vi "send_AMKSetpoint.vi"(6 "Active":bool, 7 "ID":u32=389 format="%x", 8 "Error in":errorcluster, 10 "Message":T4 {"AMK_Targetvelocity" scale=0.0..21500.0; "AMK_TorqueLimitPositive" scale=0.0..2140.0; "AMK_TorqueLimitNegative" scale=0.0..-2140.0}, 11 "ObjHandle in":T3) -> (0 "Error out":errorcluster, 3 "ObjHandle out":T3)   [LabVIEW 2017]
uses:
  <vilib>/nican/nican.llb/xobjhandle.ctl
  <vilib>/nican/nican.llb/CanFrameTimed.ctl
panel:
  in  "200/freq":i32=4
  in  "Counter":i32
  in  "CAN ID":u32=560 format="%x"
  in  "CAN frame":T1[](array[typedef]) {"Data" format="%.0x"; "ArbitrationId" format="%.0x"; "Timestamp" format="%<%I:%M:%S%3u %p\n%m/%d/%Y>T"}
  out "CAN frame out":T1[](array[typedef]) {"Data" format="%.0x"; "ArbitrationId" format="%.0x"; "Timestamp" format="%<%I:%M:%S%3u %p\n%m/%d/%Y>T"}
  in  "Message 2":T2 {"APPS2" scale=0.0..100.0; "APPS1" scale=0.0..100.0; "Steering Angle 2" scale=90.0..-90.0; "Steering Angle 1" scale=90.0..-90.0}
  in  "Active 2":bool
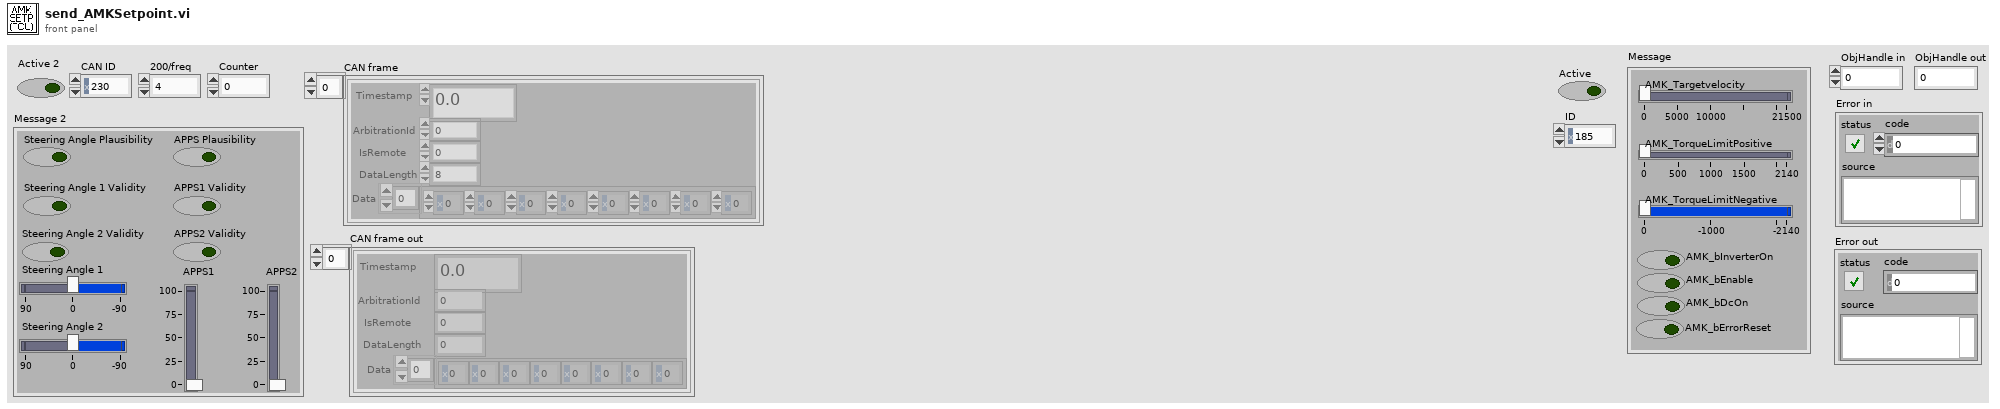
[diagram p1: front panel]
types:
  T1 = typedef "CanFrameTimed.ctl" = cluster{"Timestamp":dbl, "ArbitrationId":u32, "IsRemote":u8, "DataLength":u8, "Data":u8[]}
  T2 = cluster{"APPS Plausibility":bool, "Steering Angle 1":dbl, "Steering Angle 2":dbl, "APPS1":dbl, "APPS2":dbl, "APPS1 Validity":bool, "APPS2 Validity":bool, "Steering Angle Plausibility":bool, "Steering Angle 1 Validity":bool, "Steering Angle 2 Validity":bool}
  T3 = typedef "xobjhandle.ctl" = u32
  T4 = cluster{"AMK_bErrorReset":bool, "AMK_bDcOn":bool, "AMK_bEnable ":bool, "AMK_bInverterOn":bool, "AMK_TorqueLimitNegative":dbl, "AMK_TorqueLimitPositive":dbl, "AMK_Targetvelocity":dbl}
  T5 = cluster{"Byte 0":u8, "Byte 1":u8, "Byte 2":u8, "Byte 3":u8, "Byte 4":u8, "Byte 5":u8, "Byte 6":u8, "Byte 7":u8}
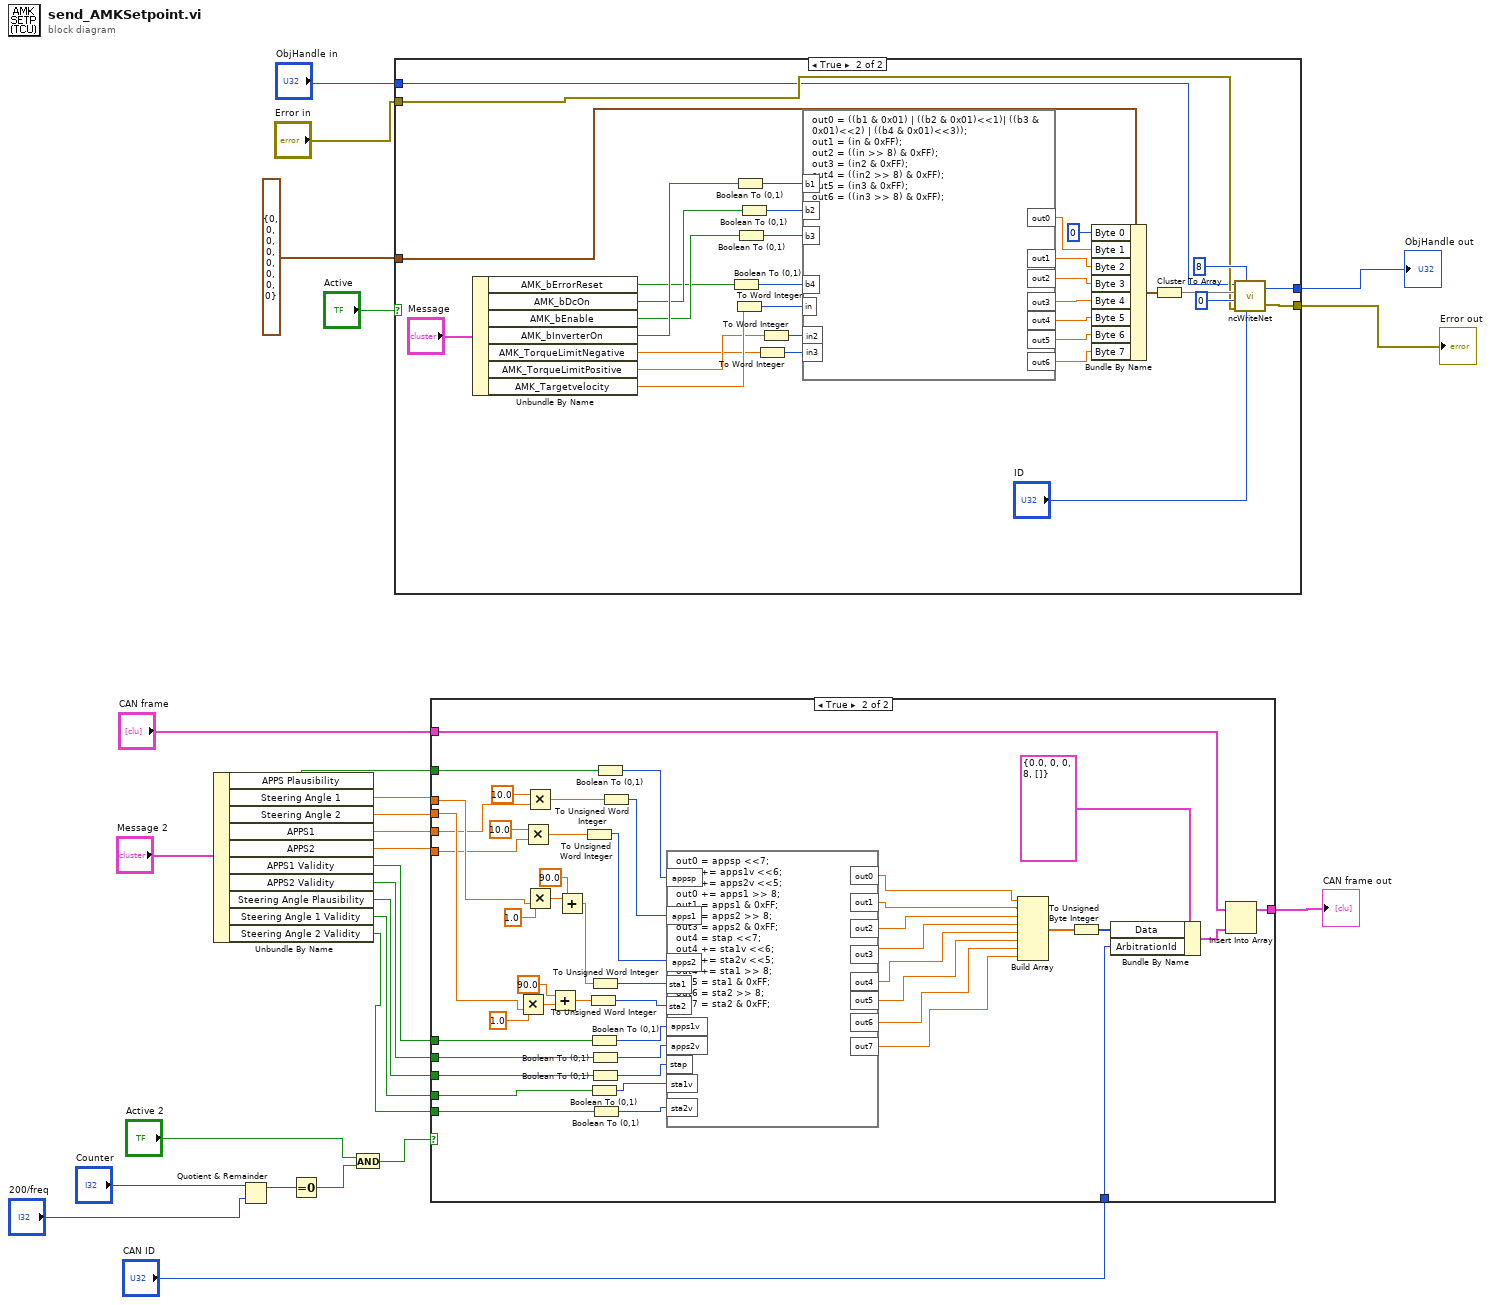
[diagram p0: block diagram]
diagram:
  n1 = Unbundle By Name("Message 2") -> ("APPS Plausibility"=w15:bool, "Steering Angle 1"=w18:dbl, "Steering Angle 2"=w19:dbl, "APPS1"=w17:dbl, "APPS2"=w16:dbl, "APPS1 Validity"=w14:bool, "APPS2 Validity"=w12:bool, "Steering Angle Plausibility"=w13:bool, "Steering Angle 1 Validity"=w11:bool, "Steering Angle 2 Validity"=w10:bool)
  n2 = Quotient & Remainder(x="Counter", y="200/freq") -> (x-y*floor(x/y)=w5:i32)  [unwired: 1 out]
  n3 = Equal To 0?(x=w5) -> (x = 0?=w3:bool)
  n4 = And(x="Active 2", y=w3) -> (x .and. y?=w2:bool)
  n5 = case shown="True" "Active" {
    tunnel: [w28 w41] -> w22
    tunnel: [w27 w40] -> w23
    tunnel: "Error in" -> [w28 w39]
    tunnel: T5 {"Byte 0"=0, "Byte 1"=0, "Byte 2"=0, "Byte 3"=0, "Byte 4"=0, "Byte 5"=0, "Byte 6"=0, "Byte 7"=0} ("CAN message") -> [_ w38]
    tunnel: "ObjHandle in" -> [w27 w37]
    frame False {
    }
    frame True {
      n6 = Unbundle By Name("Message") -> ("AMK_bErrorReset"=w32:bool, "AMK_bDcOn"=w34:bool, "AMK_bEnable"=w33:bool, "AMK_bInverterOn"=w35:bool, "AMK_TorqueLimitNegative"=w29:dbl, "AMK_TorqueLimitPositive"=w30:dbl, "AMK_Targetvelocity"=w31:dbl)
      n7 = Boolean To (0,1)(Boolean=w32) -> (0, 1=w50:i16)
      n8 = To Word Integer(number=w31) -> (16bit integer=w51:i16)
      n9 = Boolean To (0,1)(Boolean=w35) -> (0, 1=w47:i16)
      n10 = Boolean To (0,1)(Boolean=w33) -> (0, 1=w49:i16)
      n11 = Boolean To (0,1)(Boolean=w34) -> (0, 1=w48:i16)
      n12 = To Word Integer(number=w29) -> (16bit integer=w53:i16)
      n13 = To Word Integer(number=w30) -> (16bit integer=w52:i16)
      n14 = formula code="out0 = ((b1 & 0x01) | ((b2 & 0x01)<<1)| ((b3 & 0x01)<<2) | ((b4 & 0x01)<<3)); \nout1 = (in & 0xFF);\nout2 = ((in >> 8) & 0xFF);\nout3 = (in2 & 0xFF);\nout4 = ((in2 >> 8) & 0xFF);\nout5 = (in3 & 0xFF);\nout6 = ((in3 >> 8) & 0xFF);"("in"=w51, "in2"=w52, "in3"=w53, "b1"=w47, "b2"=w48, "b3"=w49, "b4"=w50) -> ("out1"=w54:dbl, "out2"=w55:dbl, "out3"=w56:dbl, "out4"=w57:dbl, "out5"=w58:dbl, "out6"=w59:dbl, "out0"=w60:dbl)
      n15 = Bundle By Name(cluster=w38, "Byte 0"=u8 0, "Byte 1"=w60, "Byte 2"=w54, "Byte 3"=w55, "Byte 4"=w56, "Byte 5"=w57, "Byte 6"=w58, "Byte 7"=w59) -> (w45:T5)
      n16 = Cluster To Array(cluster=w45) -> (array=w46:u8[])
      n17 = call <vilib>:"ncWriteNet.vi"("ArbitrationId"="ID", "DataLength"=u32 8, "Error in"=w39, "IsRemote"=u8 0, "Data"=w46, "ObjHandle in"=w37) -> ("Error out"=w41:errorcluster, "ObjHandle out"=w40:T3)
    }
  }
  "ObjHandle out" <- w23
  "Error out" <- w22
  n18 = case shown="True" w2 {
    tunnel: w19 -> [_ w93]
    tunnel: w18 -> [_ w92]
    tunnel: w17 -> [_ w91]
    tunnel: w16 -> [_ w90]
    tunnel: w15 -> [_ w89]
    tunnel: w14 -> [_ w87]
    tunnel: w13 -> [_ w86]
    tunnel: w12 -> [_ w85]
    tunnel: w11 -> [_ w84]
    tunnel: w10 -> [_ w83]
    tunnel: "CAN frame" -> [w62 w66]
    tunnel: [w62 w64] -> w8
    tunnel: "CAN ID" -> [_ w63]
    frame False {
    }
    frame True {
      n19 = Multiply(x=1.0, y=w93) -> (x*y=w103:dbl)
      n20 = Multiply(x=10.0, y=w90) -> (x*y=w100:dbl)
      n21 = Multiply(x=10.0, y=w91) -> (x*y=w101:dbl)
      n22 = Multiply(x=1.0, y=w92) -> (x*y=w105:dbl)
      n23 = Add(x=90.0, y=w103) -> (x+y=w98:dbl)
      n24 = Add(x=w105, y=90.0) -> (x+y=w99:dbl)
      n25 = To Unsigned Word Integer(number=w100) -> (unsigned 16bit integer=w95:u16)
      n26 = To Unsigned Word Integer(number=w98) -> (unsigned 16bit integer=w97:u16)
      n27 = Boolean To (0,1)(Boolean=w87) -> (0, 1=w82:i16)
      n28 = Boolean To (0,1)(Boolean=w84) -> (0, 1=w79:i16)
      n29 = To Unsigned Word Integer(number=w99) -> (unsigned 16bit integer=w96:u16)
      n30 = Boolean To (0,1)(Boolean=w85) -> (0, 1=w81:i16)
      n31 = Boolean To (0,1)(Boolean=w86) -> (0, 1=w80:i16)
      n32 = Boolean To (0,1)(Boolean=w83) -> (0, 1=w78:i16)
      n33 = Boolean To (0,1)(Boolean=w89) -> (0, 1=w88:i16)
      n34 = To Unsigned Word Integer(number=w101) -> (unsigned 16bit integer=w94:u16)
      n35 = formula code="out0 = appsp <<7;\nout0 += apps1v <<6;\nout0 += apps2v <<5;\nout0 += apps1 >> 8;\nout1 = apps1 & 0xFF;\nout2 = apps2 >> 8;\nout3 = apps2 & 0xFF;\nout4 = stap <<7;\nout4 += sta1v <<6;\nout4 += sta2v <<5;\nout4 += sta1 >> 8;\nout5 = sta1 & 0xFF;\nout6 = sta2 >> 8;\nout7 = sta2 & 0xFF;"("apps1"=w94, "apps2"=w95, "sta1"=w96, "sta2"=w97, "appsp"=w88, "apps1v"=w82, "apps2v"=w81, "stap"=w80, "sta1v"=w79, "sta2v"=w78) -> ("out1"=w76:dbl, "out2"=w75:dbl, "out3"=w74:dbl, "out0"=w77:dbl, "out4"=w73:dbl, "out5"=w72:dbl, "out6"=w71:dbl, "out7"=w70:dbl)
      n36 = Build Array(w77, w76, w75, w74, w73, w72, w71, w70) -> (w69:dbl[])
      n37 = To Unsigned Byte Integer(number=w69) -> (unsigned 8bit integer=w68:u8[])
      n38 = Bundle By Name(cluster=T1 {"Timestamp"=0.0, "ArbitrationId"=0, "IsRemote"=0, "DataLength"=8, "Data"=[]} ("CAN frame"), "Data"=w68, "ArbitrationId"=w63) -> (w65:T1)
      n39 = Insert Into Array(array=w66, new element=w65) -> (w64:T1[])  [unwired: 1 in]
    }
  }
  "CAN frame out" <- w8
